vi "Handle Error.vi"(8 "error in (no error)":errorcluster, 11 "Bob in":refnum<class "Bob.lvclass">) -> (0 "error out":errorcluster, 2 "stop actor?":bool=TRUE, 3 "Bob out":refnum<class "Bob.lvclass">)   [LabVIEW 2014, in "Bob.lvlib" / "Bob.lvclass"]
doc: "(<B>Filename</B>: Actor Framework.lvlib:Actor.lvclass:Handle Error.vi)\n\nDefines how the actor handles an error that occurred while processing a message. By default, this method does nothing except stop the actor."
uses:
  Bob.lvclass
  <vilib>/ActorFramework/Actor/Actor.lvclass
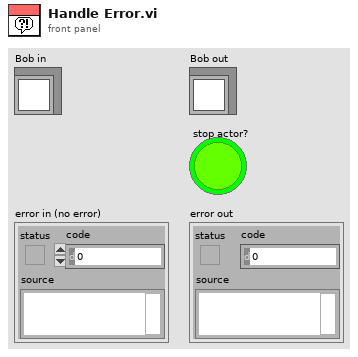
[diagram p1: front panel]
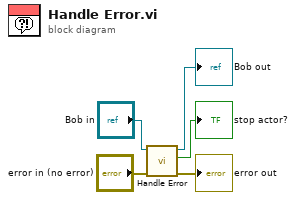
[diagram p0: block diagram]
diagram:
  n1 = call-parent "Handle Error.vi"("error in (no error)"="error in (no error)", "Actor in"="Bob in") -> ("error out"=→"error out":errorcluster, "stop actor?"=→"stop actor?":bool, "Actor out"=→"Bob out":refnum<class "Bob.lvclass">)  [unwired: 7 in]
